vi "lvEtherbone.handler_attach.vi"(0 "eb_socket_ID":i32, 2 "baseAddress":u64, 3 "maskAddress":u64, 5 "error in (no error)":errorcluster) -> (13 "eb_status":T1, 14 "eb_socket_ID out":i32, 15 "eb_handlerID":i32, 19 "error out":errorcluster)   [LabVIEW 2009, in "lvEtherbone.lvlib"]
doc: "//-----------------------------------------------------------------------------------\n// author : Dietrich Beck, GSI-Darmstadt\n// purpose : Add a device to the virtual bus.\n// This handler receives all reads and writes to the specified address.\n// the address range [0x0, 0x7fff) is reserved for internal use. \n// returns : lveb_status_t\n//-----------------------------------------------------------------------------------\nETHERBONE_API int lveb_handler_attach( int eb_socketID, //Etherbone socket ID\n eb_address_t baseAddress, //base address of THIS device\n eb_address_t maskAddress, //memory mask (range) of THIS device\n int *eb_handlerID //ID of the handler of THIS device\n );"
uses:
  lvEtherbone.lvlib
  lvEtherbone.lveb_status_t.ctl
  bin/lvEtherbone.dll
panel:
  in  "myeb_status_t":T1
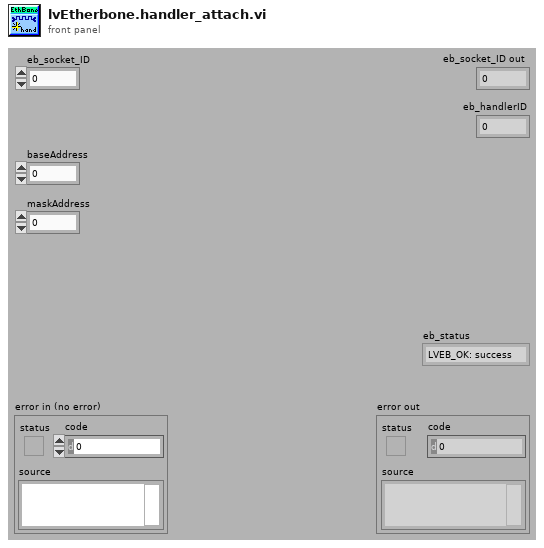
[diagram p1: front panel]
types:
  T1 = typedef "lvEtherbone.lvlib/lvEtherbone.lveb_status_t.ctl" = enum32{"LVEB_OK: success", "LVEB_UNKNOWN: unknown error", "LVEB_OS: operating system forbids access", "LVEB_PORT: port in use or unavailable", "LVEB_ID: ID invalid or out of resources", "LVEB_SOCKET: socket invalid or unavailable", "LVEB_EB: remote address is not Etherbone conformant", "LVEB_IP: bad format or network address", "LVEB_PORTWIDTH: port width error", "LVEB_DEVICEBUSY: Etherbone device still busy", "LVEB_DEVICEFAIL: operation on Wishbone device failed", "LVEB_DEVICEEXIST: Etherbone device already exists, overlaps, or does not exist", "LVEB_TIMEDOUT: a timeout occurred", "LVEB_OVERFLOW: payload of Etherbone exceeded", "LVEB_ADDRESS: bad address", "LVEB_ADDRESSWIDTH: address width error"}
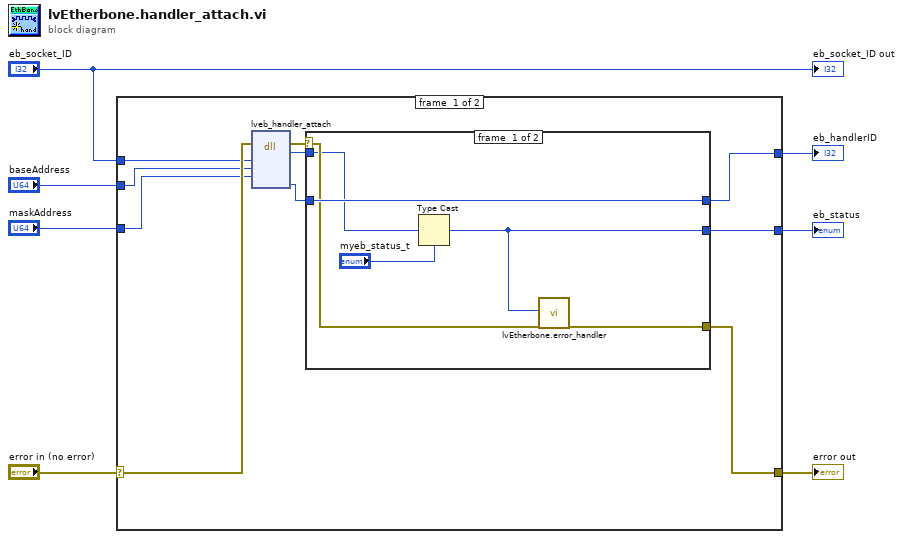
[diagram p0: block diagram]
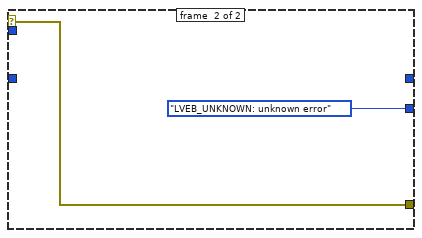
[diagram p2: hidden frame]
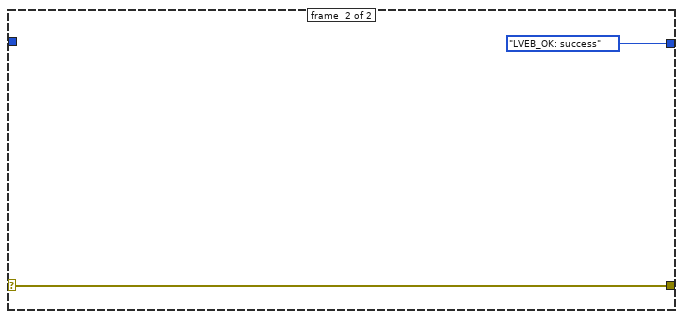
[diagram p3: hidden frame]
diagram:
  n1 = case shown="No Error" "error in (no error)" {
    selector: "error in (no error)" -> [w17 w27]
    tunnel: [w12 w27] -> w6
    tunnel: "eb_socket_ID" -> [w16 _]
    tunnel: "baseAddress" -> [w15 _]
    tunnel: [w10 lvEtherbone.lveb_status_t."LVEB_OK: success" ("eb_status_t")] -> w4
    tunnel: [w11 _] -> w1
    tunnel: "maskAddress" -> [w9 _]
    frame #0 {
      n2 = dll-call lib="F:/beck/Project/BEL/SCC/etherbone-core/api/lvEtherbone/bin/lvEtherbone.*" fn="lveb_handler_attach"(error in=w17, "eb_socketID"=w16, "baseAddress"=w15, "maskAddress"=w9) -> (error out=w14:errorcluster, "myeb_status"=w13:i32, "eb_handlerID"=w8:i32)  [unwired: 6 in, 1 out]
      n3 = case shown="Error" w14 {
        selector: w14 -> [w21 w25]
        tunnel: w13 -> [w20 _]
        tunnel: [w19 lvEtherbone.lveb_status_t."LVEB_UNKNOWN: unknown error" ("eb_status_t")] -> w10
        tunnel: [w22 w25] -> w12
        tunnel: w8 -> [w23 _]
        tunnel: [w23 _] -> w11
        frame #0 {
          n4 = Type Cast(type="myeb_status_t", x=w20) -> (*(type *) &x=w19:T1)
          n5 = call "lvEtherbone.error_handler.vi"("eb_status"=w19, "error in"=w21) -> ("error out"=w22:errorcluster)  [unwired: 17 in]
        }
        frame #1 {
        }
      }
    }
    frame #1 {
    }
  }
  "error out" <- w6
  "eb_status" <- w4
  "eb_handlerID" <- w1
  "eb_socket_ID out" <- "eb_socket_ID"
